vi "ELVIS III v1.0 Build MUX Configuration AI.vi"(11 "AI Channels List":T4) -> (3 "Channel Reservation Info":T1)   [LabVIEW 2021]
uses:
  <vilib>/myRIO/Common/Instrument Driver Framework/myRIO v1.0/AI/typedefs/AI Channels List.ctl
  <vilib>/myRIO/Common/Instrument Driver Framework/myRIO v1.0/AI/typedefs/AI Channels Enum.ctl
  <vilib>/myRIO/Common/Instrument Driver Framework/ELVIS III v1.0/Resource Manager/typedefs/ELVIS III v1.0 Channel Reservation List.ctl
  <vilib>/myRIO/Common/Instrument Driver Framework/ELVIS III v1.0/Resource Manager/typedefs/ELVIS III v1.0 Channel Reservation Info.ctl
  <vilib>/myRIO/Common/Instrument Driver Framework/ELVIS III v1.0/Resource Manager/typedefs/ELVIS III v1.0 Connector List.ctl
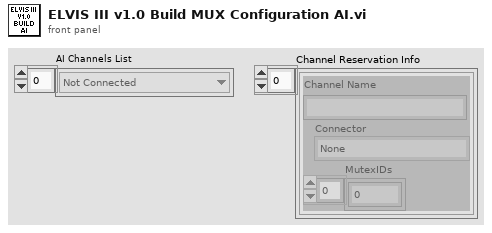
[diagram p1: front panel]
types:
  T1 = typedef "ELVIS III v1.0 Channel Reservation List.ctl" = T2[]
  T2 = typedef "ELVIS III v1.0 Channel Reservation Info.ctl" = cluster{"Channel Name":string, "Connector":T3, "MutexIDs":u32[]}
  T3 = typedef "ELVIS III v1.0 Connector List.ctl" = enum32{"None", "ConnectorA", "ConnectorB"}
  T4 = typedef "AI Channels List.ctl" = T5[]
  T5 = typedef "AI Channels Enum.ctl" = enum16{"Not Connected", "AudioIn/Left", "AudioIn/Right", "C/AI0", "C/AI1", "A/AI0", "A/AI1", "A/AI2", "A/AI3", "A/AI4", "A/AI5", "A/AI6", "A/AI7", "B/AI0", "B/AI1", "B/AI2", "B/AI3", "B/AI4", "B/AI5", "B/AI6", "B/AI7", "AI/AI0", "AI/AI1", "AI/AI2", "AI/AI3", "A/AI0 (DIFF)", "A/AI1 (DIFF)", "A/AI2 (DIFF)", "A/AI3 (DIFF)", "B/AI0 (DIFF)", "B/AI1 (DIFF)", "B/AI2 (DIFF)", "B/AI3 (DIFF)"}
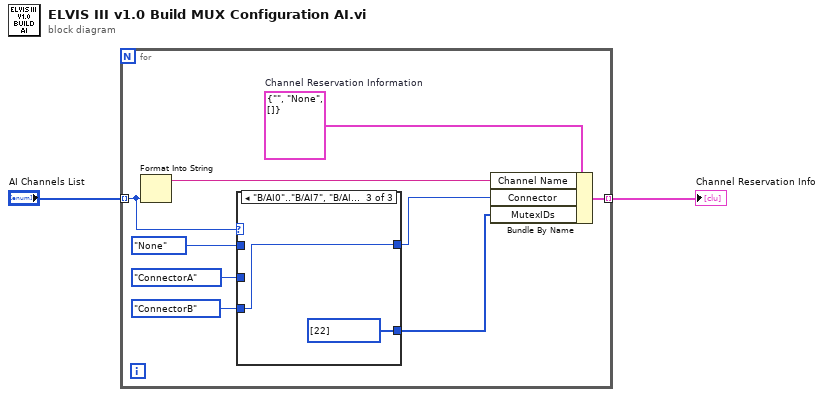
[diagram p0: block diagram]
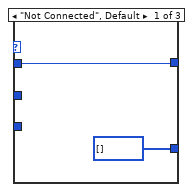
[diagram p2: hidden frame]
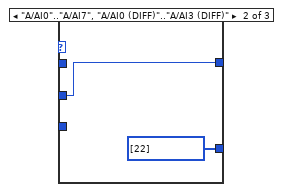
[diagram p3: hidden frame]
diagram:
  n1 = for {
    tunnel: "AI Channels List" -> [w8] mode=indexing
    tunnel: [w9] -> w1 mode=indexing
    w11 = T2 {"Channel Name"="", "Connector"=enum."None", "MutexIDs"=[]}  # Channel Reservation Information
    n2 = Format Into String(w8) -> (resulting string=w10:string)  [unwired: 3 in, 1 out]
    n3 = case shown="\"B/AI0\"..\"B/AI7\", \"B/AI0 (DIFF)\"..\"B/AI3 (DIFF)\"" w8 {
      tunnel: [u32[] [] ("MutexIDs") u32[] [22] ("MutexIDs") u32[] [22] ("MutexIDs")] -> w7
      tunnel: ELVIS_III_v1.0_Connector_List."None" ("Connector") -> [w13 _ _]
      tunnel: [w13 w15 w16] -> w5
      tunnel: ELVIS_III_v1.0_Connector_List."ConnectorA" ("Connector") -> [_ w15 _]
      tunnel: ELVIS_III_v1.0_Connector_List."ConnectorB" ("Connector") -> [_ _ w16]
      frame "Not Connected", Default {
      }
      frame "A/AI0".."A/AI7", "A/AI0 (DIFF)".."A/AI3 (DIFF)" {
      }
      frame "B/AI0".."B/AI7", "B/AI0 (DIFF)".."B/AI3 (DIFF)" {
      }
    }
    n4 = Bundle By Name(cluster=w11, "Channel Name"=w10, "Connector"=w5, "MutexIDs"=w7) -> (w9:T2)
  }
  "Channel Reservation Info" <- w1
